vi "Spreadsheet Storage (OpenWriteClose).vi"() -> ()   [LabVIEW 2015]
panel:
  in  "Waveform Parameters":T1
  in  "Digitizing Parameters":T2
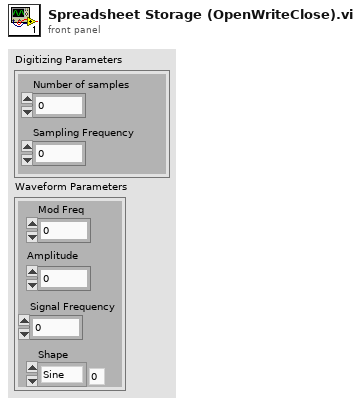
[diagram p1: front panel]
types:
  T1 = cluster{"Mod Freq":dbl, "Amplitude":dbl, "Shape":enum16{"Sine", "Cosine", "DC Level", "Square", "User Defined"}, "Signal Frequency":dbl}
  T2 = cluster{"Number of samples":dbl, "Sampling Frequency":dbl}
  T3 = enum16{"open", "replace", "create", "open or create", "replace or create", "replace or create with confirmation"}
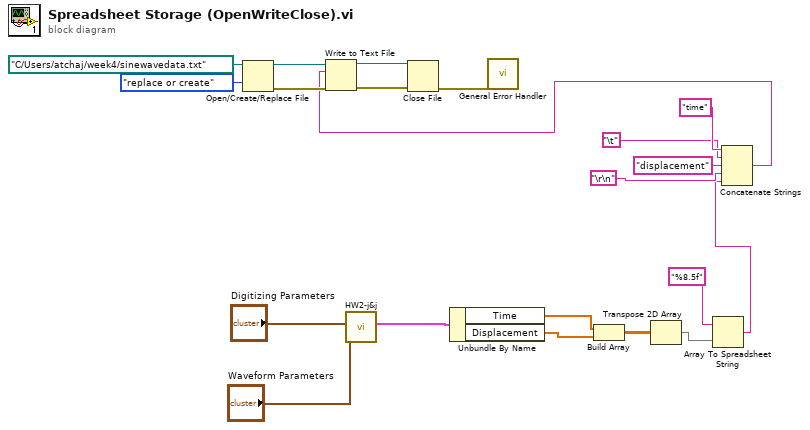
[diagram p0: block diagram]
diagram:
  n1 = Open/Create/Replace File(file path (use dialog)=path "C:/Users/atchaj/week4/sinewavedata.txt", operation (0:open)=T3."replace or create") -> (refnum out=w12:refnum<file>, error out=w13:errorcluster)  [unwired: 4 in, 1 out]
  n2 = call "HW2-j&j.vi"("AM Wave Parameters"="Waveform Parameters", "Digitizing Parameters"="Digitizing Parameters") -> ("AM Wave"=w21:cluster{"Time":dbl[], "Displacement":dbl[]})  [unwired: 9 in]
  n3 = Unbundle By Name(w21) -> ("Time"=w18:dbl[], "Displacement"=w17:dbl[])
  n4 = Build Array(w18, w17) -> (w7:dbl[][])
  n5 = Transpose 2D Array(2D array=w7) -> (transposed array=w8:dbl[][])
  n6 = Array To Spreadsheet String(array=w8, 3:"%8.5f" ("format string")) -> (spreadsheet string=w2:string)  [unwired: 1 in]
  n7 = Concatenate Strings("time" ("string"), "\t", "displacement" ("string"), "\r\n", w2) -> (w1:string)
  n8 = Write to Text File(file (use dialog)=w12, text=w1, error in=w13) -> (refnum out=w11:refnum<file>, error out=w14:errorcluster)  [unwired: 1 in, 1 out]
  n9 = Close File(refnum=w11, error in=w14) -> (error out=w15:errorcluster)  [unwired: 1 out]
  n10 = call <vilib>:"General Error Handler.vi"("error in (no error)"=w15) -> ()  [unwired: 10 in, 5 out]
